vi "String To Number(I32).vi"(5 "String":string) -> (0 "Numeric(I32)":i32)   [LabVIEW 2017]
uses:
  <userlib>/_OpenG.lib/string/string.llb/Trim Whitespace (String)__ogtk.vi
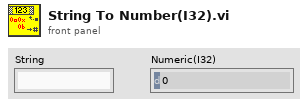
[diagram p1: front panel]
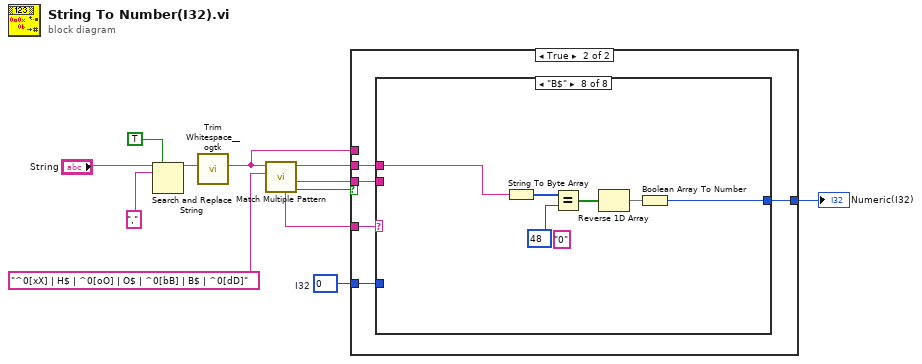
[diagram p0: block diagram]
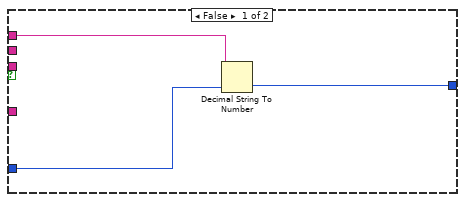
[diagram p2: hidden frame]
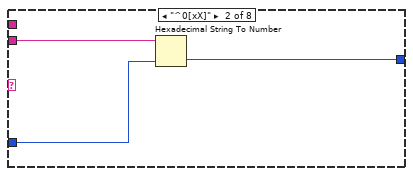
[diagram p4: hidden frame]
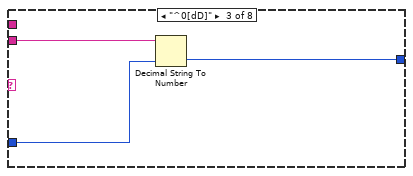
[diagram p5: hidden frame]
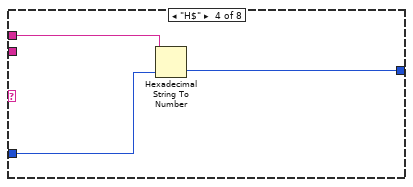
[diagram p6: hidden frame]
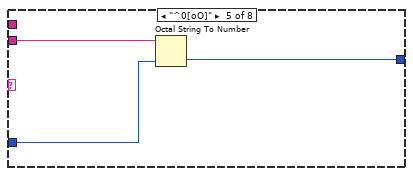
[diagram p7: hidden frame]
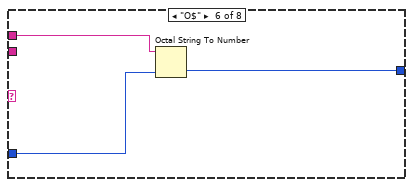
[diagram p8: hidden frame]
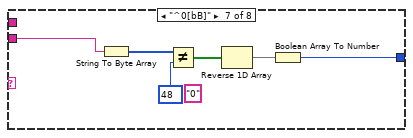
[diagram p9: hidden frame]
diagram:
  w1 = 0  # I32
  n1 = Search and Replace String(replace all?=TRUE ("replace all? (F)"), input string="String", search string=",") -> (result string=w9:string)  [unwired: 5 in, 3 out]
  n2 = call-poly <userlib>:"Trim Whitespace__ogtk.vi"("String in"=w9) -> ("String out"=w2:string)  [unwired: 6 in]
  n3 = call "Match Multiple Pattern.vi"("regular expression"="^0[xX] | H$ | ^0[oO] | O$ | ^0[bB] | B$ | ^0[dD]", "string"=w2) -> ("Found?"=w7:bool, "after substring"=w5:string, "before substring"=w4:string, "pattern matched"=w6:string)  [unwired: 5 in, 1 out]
  n4 = case shown="True" w7 {
    tunnel: w6 -> [_ w20]
    tunnel: w5 -> [_ w19]
    tunnel: w4 -> [_ w18]
    tunnel: [w15 w17] -> w3
    tunnel: w2 -> [w14 _]
    tunnel: w1 -> [w13 w16]
    frame False {
      n5 = Decimal String To Number(string=w14, default (0L)=w13) -> (number=w15:i32)  [unwired: 1 in, 1 out]
    }
    frame True {
      n6 = case shown="\"B$\"" w20 {
        tunnel: w19 -> [_ w24 w27 _ w33 _ w41 _]
        tunnel: w18 -> [_ _ _ w29 _ w35 _ w45]
        tunnel: [w21 w23 w26 w30 w32 w36 w42 w48] -> w17
        tunnel: w16 -> [w21 w22 w25 w28 w31 w34 _ _]
        frame Default {
        }
        frame "^0[xX]" {
          n7 = Hexadecimal String To Number(string=w24, default (0uL)=w22) -> (number=w23:i32)  [unwired: 1 in, 1 out]
        }
        frame "^0[dD]" {
          n8 = Decimal String To Number(string=w27, default (0L)=w25) -> (number=w26:i32)  [unwired: 1 in, 1 out]
        }
        frame "H$" {
          n9 = Hexadecimal String To Number(string=w29, default (0uL)=w28) -> (number=w30:i32)  [unwired: 1 in, 1 out]
        }
        frame "^0[oO]" {
          n10 = Octal String To Number(2:w31, 4:w33) -> (0:w32:i32)  [unwired: 1 in, 1 out]
        }
        frame "O$" {
          n11 = Octal String To Number(2:w34, 4:w35) -> (0:w36:i32)  [unwired: 1 in, 1 out]
        }
        frame "^0[bB]" {
          (unwired) "0" ("search string")
          n12 = String To Byte Array(string=w41) -> (unsigned byte array=w40:u8[])
          n13 = Not Equal?(x=w40, y=u8 48) -> (x != y?=w38:bool[])
          n14 = Reverse 1D Array(array=w38) -> (reversed array=w37:bool[])
          n15 = Boolean Array To Number(Boolean array=w37) -> (number=w42:i32)
        }
        frame "B$" {
          (unwired) "0" ("search string")
          n16 = String To Byte Array(string=w45) -> (unsigned byte array=w47:u8[])
          n17 = Equal?(x=w47, y=u8 48) -> (x = y?=w46:bool[])
          n18 = Reverse 1D Array(array=w46) -> (reversed array=w44:bool[])
          n19 = Boolean Array To Number(Boolean array=w44) -> (number=w48:i32)
        }
      }
    }
  }
  "Numeric(I32)" <- w3
